vi "New.vi"(8 "Error In":errorcluster, 11 "Content":string) -> (0 "Error Out":errorcluster, 3 "Text":refnum<class "Text.lvclass">)   [LabVIEW 2018, in "Toolkit.lvlib" / "Tokens.lvlib" / "Text.lvclass"]
uses:
  Text.lvclass
  Text.lvclass/Text.ctl
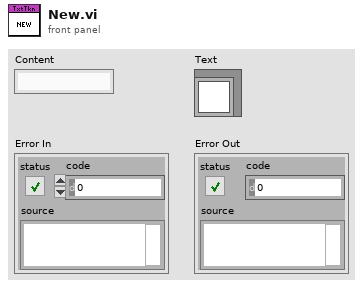
[diagram p1: front panel]
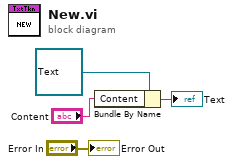
[diagram p0: block diagram]
diagram:
  n1 = Bundle By Name(cluster=refnum<class "Text.lvclass"> refnum ("Mustache.lvlib:Tokens.lvlib:Text.lvclass"), "Content"="Content") -> (→"Text":refnum<class "Text.lvclass">)
  "Error Out" <- "Error In"
